vi "Untitled 1.vi"(2 "Lado C":dbl, 3 "Lado B":dbl, 4 "Lado A":dbl) -> (0 "Triangulo Invalido":bool, 1 "Area":dbl)   [LabVIEW 2016]
doc: "Este VI se dedica a calcualar el area de un traingulo dandonde los tres lados e indica si dicho traingulo es valido o no"
panel:
  out "error out":errorcluster
  in  "error in (no error)":errorcluster
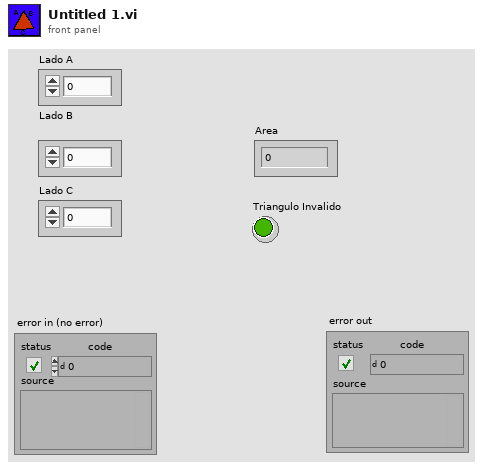
[diagram p1: front panel]
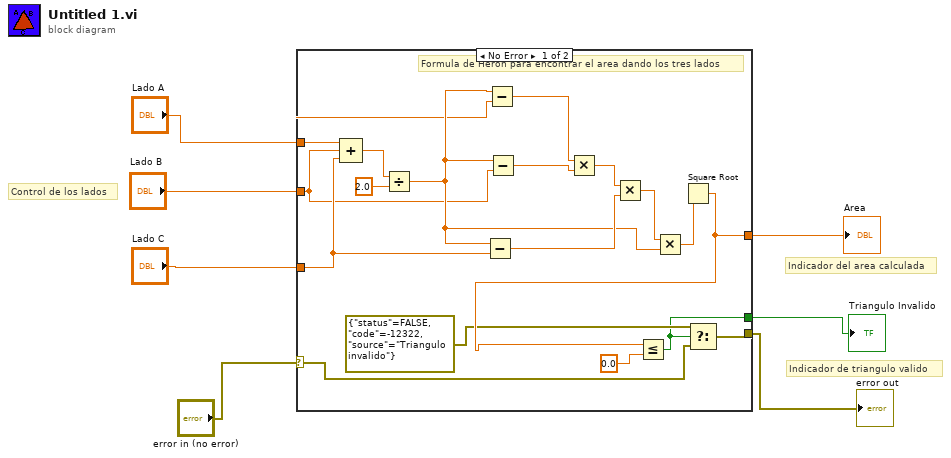
[diagram p0: block diagram]
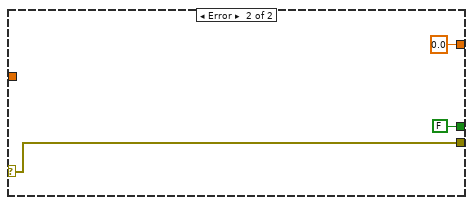
[diagram p2: hidden frame]
diagram:
  # "Control de los lados"
  # "Indicador del area calculada"
  # "Indicador de triangulo valido"
  n1 = case shown="No Error" "error in (no error)" {
    selector: "error in (no error)" -> [w10 w28]
    tunnel: "Lado C" -> [w23 _]
    tunnel: "Lado A" -> [w15 _]
    tunnel: "Lado B" -> [w14 _]
    tunnel: [w12 0.0] -> w4
    tunnel: [w11 w28] -> w2
    tunnel: [w8 FALSE] -> w1
    frame No Error {
      # "Formula de Heron para encontrar el area dando los tres lados"
      n2 = Compound Arithmetic op=ADD(w15, w14, w23) -> (w25:dbl)
      n3 = Divide(x=w25, y=2.0) -> (x/y=w17:dbl)
      n4 = Subtract(x=w17, y=w23) -> (x-y=w19:dbl)
      n5 = Subtract(x=w17, y=w15) -> (x-y=w22:dbl)
      n6 = Subtract(x=w17, y=w14) -> (x-y=w21:dbl)
      n7 = Multiply(x=w22, y=w21) -> (x*y=w20:dbl)
      n8 = Multiply(x=w20, y=w19) -> (x*y=w18:dbl)
      n9 = Multiply(x=w18, y=w17) -> (x*y=w16:dbl)
      n10 = Square Root(x=w16) -> (sqrt(x)=w12:dbl)
      n11 = Less Or Equal?(x=w12, y=0.0) -> (x <= y?=w8:bool)
      n12 = Select(t=errorcluster {"status"=FALSE, "code"=-12322, "source"="Triangulo invalido"} ("error constant"), s=w8, f=w10) -> (s? t:f=w11:errorcluster)
    }
    frame Error {
    }
  }
  "Area" <- w4
  "Triangulo Invalido" <- w1
  "error out" <- w2
